vi "Unflatten Value.vi"(8 "error in (no error)":errorcluster, 10 "Value":string, 11 "Boolean in":refnum<class "Path Builder.lvclass">) -> (0 "error out":errorcluster, 3 "Boolean out":refnum<class "Path Builder.lvclass">)   [LabVIEW 2017, in "Custom Type Test Executive.lvlib" / "Path Builder.lvclass"]
uses:
  <vilib>/gpm_packages/@cs/test-executive/Source/Custom Type Test Executive/Path Builder Data Type/Path Builder.lvclass
  <vilib>/gpm_packages/@cs/test-executive/Source/Path Builder/IPath Builder/IPath Builder.lvclass
  <vilib>/gpm_packages/@cs/test-executive/Source/Custom Type Test Executive/Path Builder Data Type/Path Builder.lvclass/Path Builder.ctl
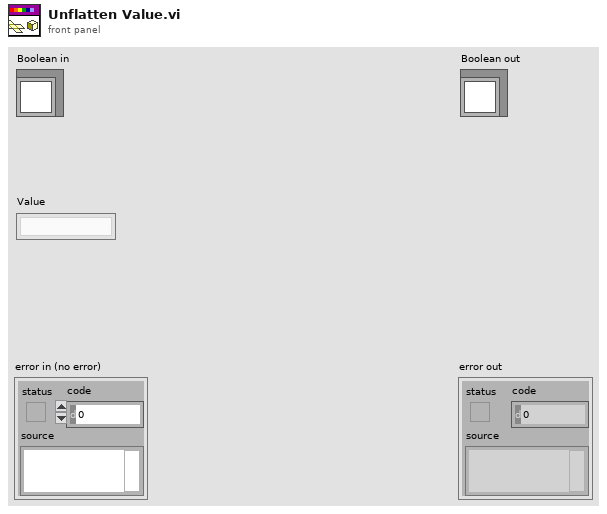
[diagram p1: front panel]
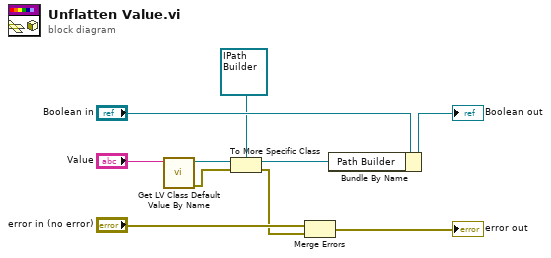
[diagram p0: block diagram]
diagram:
  n1 = call <vilib>:"Get LV Class Default Value By Name.vi"("class name"="Value") -> ("error out"=w2:errorcluster, "object"=w6:refnum<class>)  [unwired: 9 in]
  n2 = To More Specific Class(target class=refnum<class "IPath Builder.lvclass"> refnum ("Path Builder"), reference=w6, error in=w2) -> (specific class reference=w5:refnum<class "IPath Builder.lvclass">, error out=w3:errorcluster)
  n3 = Merge Errors("error in (no error)", w3) -> (→"error out":errorcluster)
  n4 = Bundle By Name(cluster="Boolean in", "Path Builder"=w5) -> (→"Boolean out":refnum<class "Path Builder.lvclass">)
